vi "Item_OnCommand.vi"(10 "Command ID":string, 11 "Item Ref":T1) -> ()   [LabVIEW 2020, in "Negentropic IDE.lvlib"]
uses:
  Negentropic IDE.lvlib
  <resource>/Framework/Providers/API/ItemRef.ctl
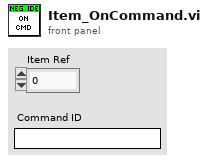
[diagram p1: front panel]
types:
  T1 = typedef "ItemRef.ctl" = u64
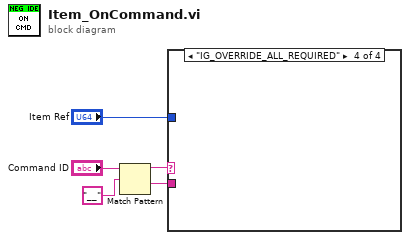
[diagram p0: block diagram]
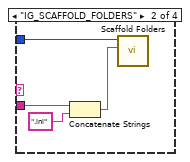
[diagram p3: hidden frame]
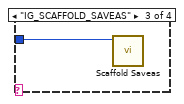
[diagram p4: hidden frame]
diagram:
  n1 = Match Pattern(string="Command ID", regular expression="__") -> (before substring=w2:string, after substring=w1:string)  [unwired: 1 in, 2 out]
  n2 = case shown="\"IG_OVERRIDE_ALL_REQUIRED\"" w2 {
    tunnel: "Item Ref" -> [_ w9 w10 _]
    tunnel: w1 -> [_ w8 _ _]
    frame Default {
    }
    frame "IG_SCAFFOLD_FOLDERS" {
      n3 = Concatenate Strings(w8, ".ini" ("string")) -> (w6:string)
      n4 = call "Scaffold Folders.vi"("INI Filename"=w6, "Item Ref"=w9) -> ()  [unwired: 10 in]
    }
    frame "IG_SCAFFOLD_SAVEAS" {
      n5 = call "Scaffold Saveas.vi"("Item Ref"=w10) -> ()  [unwired: 11 in]
    }
    frame "IG_OVERRIDE_ALL_REQUIRED" {
    }
  }
